vi "zadanie3_kol.vi"() -> ()   [LabVIEW 2012]
panel:
  in  "Wybierz jednostkê czêstotliwoœci drgañ:":u16(ring) items=["giga herc", "herc", "mili herc", "mikro herc"]
  out "Czêstotliwoœæ (w wybranej jednostce):":dbl
  in  "Okres drgañ (w wybranej jednostce)":dbl
  in  "Wybierz jednostkê okresu drgañ":u16(ring) items=["minuty", "sekundy", "milisekundy", "mikrosekundy"]
  # "Program oblicza czêstotliwoœæ na podstawie podanego okresu drgañ\noraz pozwala na zmianê jednostek okresu drgañ i czêstotliwoœci"
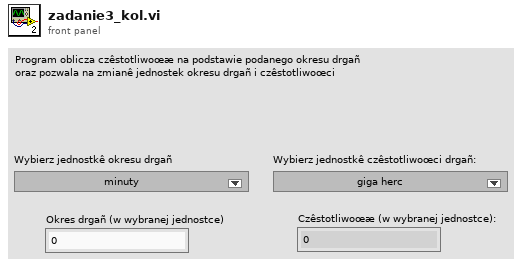
[diagram p1: front panel]
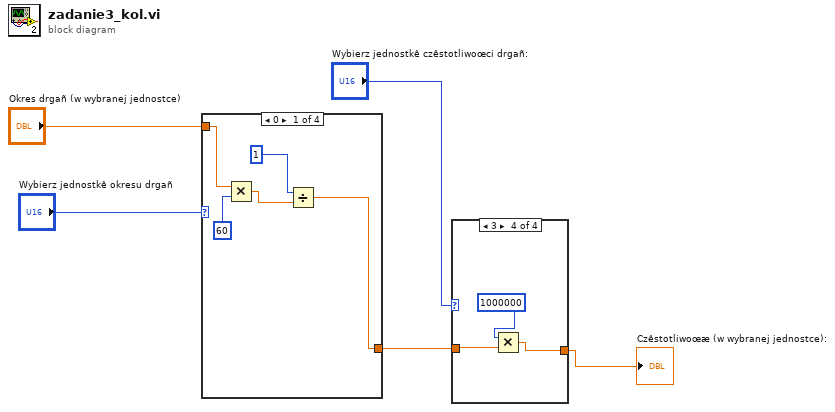
[diagram p0: block diagram]
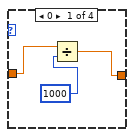
[diagram p2: hidden frame]
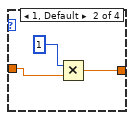
[diagram p3: hidden frame]
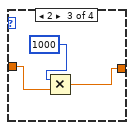
[diagram p4: hidden frame]
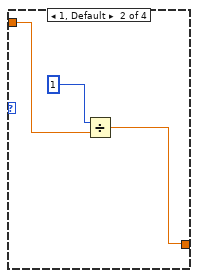
[diagram p5: hidden frame]
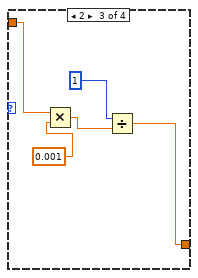
[diagram p6: hidden frame]
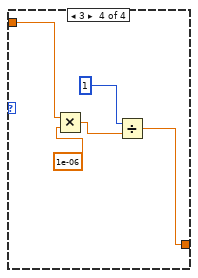
[diagram p7: hidden frame]
diagram:
  n1 = case shown="0" "Wybierz jednostkê okresu drgañ" {
    tunnel: "Okres drgañ (w wybranej jednostce)" -> [w9 w12 w16 w20]
    tunnel: [w6 w11 w14 w19] -> w2
    frame 0 {
      n2 = Multiply(x=w9, y=60) -> (x*y=w8:dbl)
      n3 = Divide(x=1, y=w8) -> (x/y=w6:dbl)
    }
    frame 1, Default {
      n4 = Divide(x=1, y=w12) -> (x/y=w11:dbl)
    }
    frame 2 {
      n5 = Multiply(x=w16, y=0.001) -> (x*y=w17:dbl)
      n6 = Divide(x=1, y=w17) -> (x/y=w14:dbl)
    }
    frame 3 {
      n7 = Multiply(x=w20, y=1e-06) -> (x*y=w22:dbl)
      n8 = Divide(x=1, y=w22) -> (x/y=w19:dbl)
    }
  }
  n9 = case shown="3" "Wybierz jednostkê czêstotliwoœci drgañ:" {
    tunnel: w2 -> [w26 w28 w32 w34]
    tunnel: [w24 w27 w30 w33] -> w1
    frame 0 {
      n10 = Divide(x=w26, y=1000) -> (x/y=w24:dbl)
    }
    frame 1, Default {
      n11 = Multiply(x=1, y=w28) -> (x*y=w27:dbl)
    }
    frame 2 {
      n12 = Multiply(x=1000, y=w32) -> (x*y=w30:dbl)
    }
    frame 3 {
      n13 = Multiply(x=1000000, y=w34) -> (x*y=w33:dbl)
    }
  }
  "Czêstotliwoœæ (w wybranej jednostce):" <- w1
